vi "createTable sortie ROI.vi"() -> ()   [LabVIEW 2019]
panel:
  out "R7 chiffre":string
  out "R1 chiffre":string
  out "R4 chiffre":string
  out "Y3 chiffre":string
  out "Y1 chiffre":string
  out "Y2 chiffre":string
  out "G6 chiffre":string
  out "G9 chiffre":string
  out "Y7 chiffre":string
  out "R2 chiffre":string
  out "Y4 chiffre":string
  out "G3 chiffre":string
  out "G7 chiffre":string
  out "O3 chiffre":string
  out "G2 chiffre":string
  out "O9 chiffre":string
  out "W7 chiffre":string
  out "W8 chiffre":string
  out "W9 chiffre":string
  out "G8 chiffre":string
  out "G4 chiffre":string
  out "O6 chiffre":string
  out "G1 chiffre":string
  out "W6 chiffre":string
  out "O2 chiffre":string
  out "O1 chiffre":string
  out "O8 chiffre":string
  out "O7 chiffre":string
  out "O4 chiffre":string
  out "Y6 chiffre":string
  out "Y8 chiffre":string
  out "Y9 chiffre":string
  out "B7 chiffre":string
  out "B4 chiffre":string
  out "R8 chiffre":string
  out "B2 chiffre":string
  out "W4 chiffre":string
  out "R9 chiffre":string
  out "B8 chiffre":string
  out "B9 chiffre":string
  out "B6 chiffre":string
  out "R3 chiffre":string
  out "B3 chiffre":string
  out "B1 chiffre":string
  out "W3 chiffre":string
  out "R6 chiffre":string
  out "W2 chiffre":string
  out "W1 chiffre":string
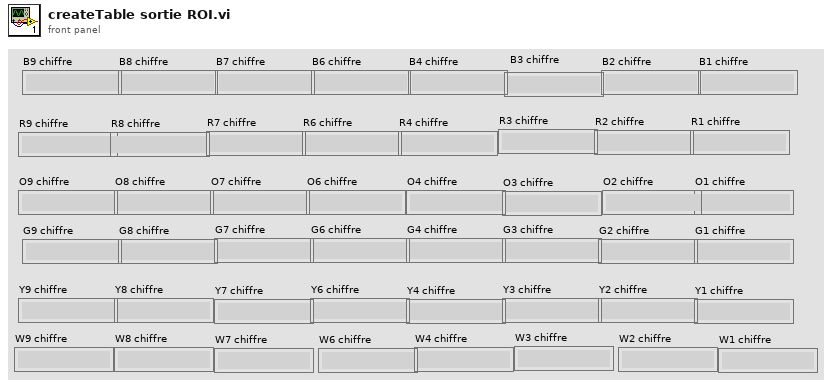
[diagram p1: front panel]
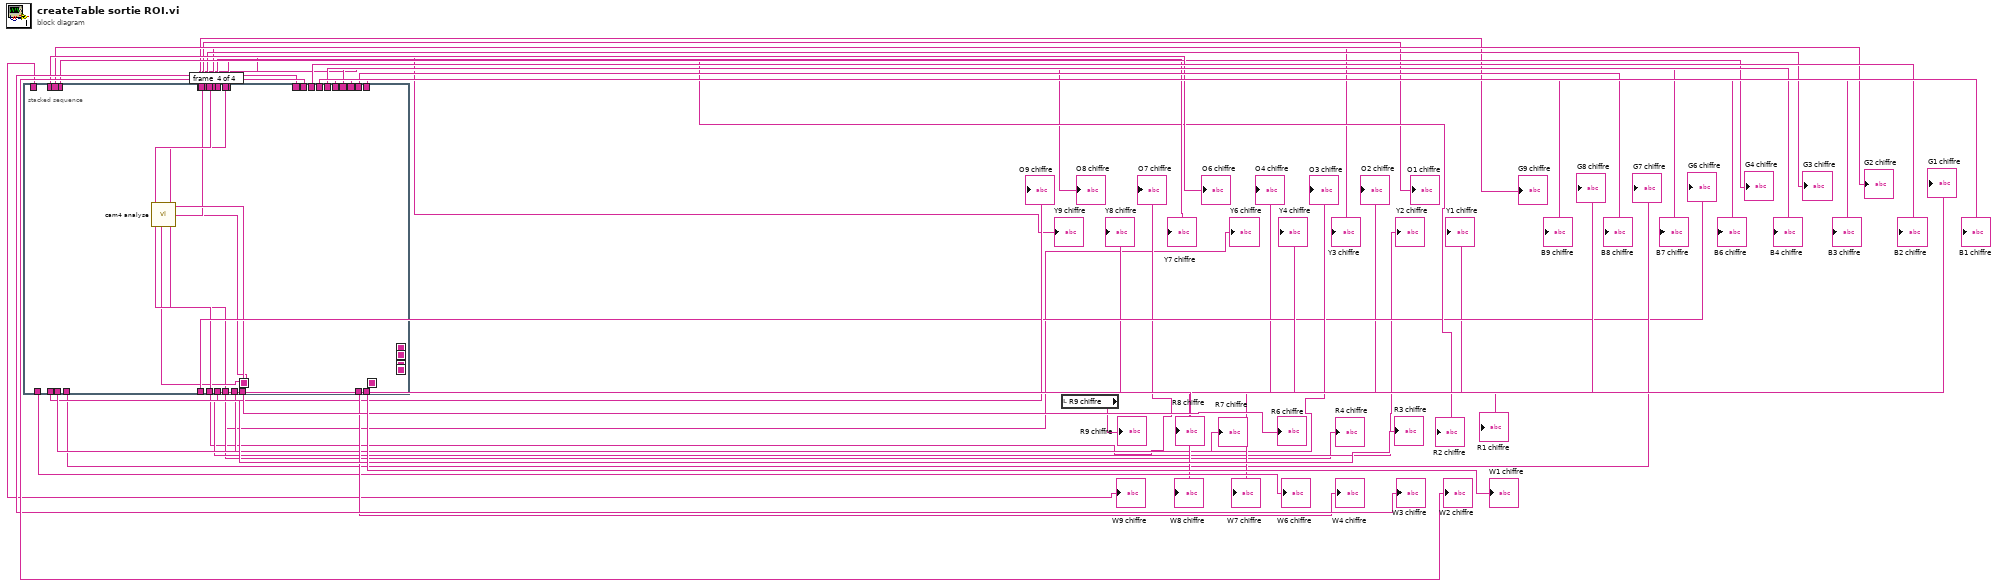
[diagram p0: block diagram]
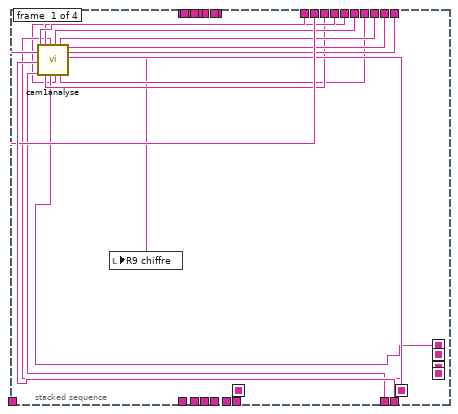
[diagram p2: hidden frame]
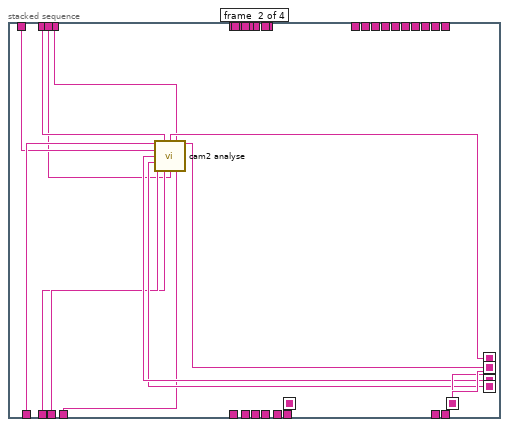
[diagram p3: hidden frame]
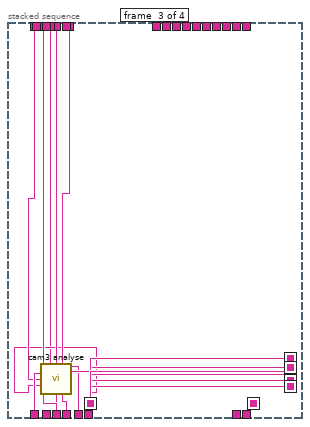
[diagram p4: hidden frame]
diagram:
  n1 = stacked-sequence {
    seq-local: [w62 _ _ _] -> [_ w79 _ _]
    seq-local: [w58 _ _ _] -> [_ w78 _ _]
    seq-local: [w52 _ _ _] -> [_ w77 _ _]
    seq-local: [_ w79 _ _] -> [_ _ w98 _]
    seq-local: [_ w78 _ _] -> [_ _ w97 _]
    seq-local: [_ w77 _ _] -> [_ _ w96 _]
    seq-local: [_ w74 _ _] -> [_ _ w95 _]
    seq-local: [_ w72 _ _] -> [_ _ w94 _]
    seq-local: [_ w70 _ _] -> [_ _ w93 _]
    seq-local: [_ w69 _ _] -> [_ _ w92 _]
    seq-local: [_ _ w98 _] -> [_ _ _ w115]
    seq-local: [_ _ w97 _] -> [_ _ _ w114]
    seq-local: [_ _ w96 _] -> [_ _ _ w113]
    seq-local: [_ _ w95 _] -> [_ _ _ w112]
    seq-local: [_ _ w94 _] -> [_ _ _ w111]
    seq-local: [_ _ w93 _] -> [_ _ _ w110]
    seq-local: [_ _ w92 _] -> [_ _ _ w109]
    seq-local: [_ _ w90 _] -> [_ _ _ w108]
    seq-local: [_ _ w84 _] -> [_ _ _ w107]
    tunnel: [w64 _ _ _] -> w48
    tunnel: [w63 _ _ _] -> w47
    tunnel: [w61 _ _ _] -> w45
    tunnel: [w60 _ _ _] -> w44
    tunnel: [w59 _ _ _] -> w43
    tunnel: [w57 _ _ _] -> w41
    tunnel: [w56 _ _ _] -> w40
    tunnel: [w55 _ _ _] -> w39
    tunnel: [w54 _ _ _] -> w38
    tunnel: [w53 _ _ _] -> w37
    tunnel: [w51 _ _ _] -> w35
    tunnel: [w50 _ _ _] -> w34
    tunnel: [_ w76 _ _] -> w33
    tunnel: [_ w75 _ _] -> w32
    tunnel: [_ w73 _ _] -> w30
    tunnel: [_ w71 _ _] -> w28
    tunnel: [_ w68 _ _] -> w25
    tunnel: [_ w67 _ _] -> w24
    tunnel: [_ w66 _ _] -> w23
    tunnel: [_ w65 _ _] -> w22
    tunnel: [_ _ w91 _] -> w21
    tunnel: [_ _ w89 _] -> w19
    tunnel: [_ _ w88 _] -> w18
    tunnel: [_ _ w87 _] -> w17
    tunnel: [_ _ w86 _] -> w16
    tunnel: [_ _ w85 _] -> w15
    tunnel: [_ _ w83 _] -> w13
    tunnel: [_ _ w82 _] -> w12
    tunnel: [_ _ w81 _] -> w11
    tunnel: [_ _ w80 _] -> w10
    tunnel: [_ _ _ w115] -> w46
    tunnel: [_ _ _ w114] -> w42
    tunnel: [_ _ _ w113] -> w36
    tunnel: [_ _ _ w112] -> w31
    tunnel: [_ _ _ w111] -> w29
    tunnel: [_ _ _ w110] -> w27
    tunnel: [_ _ _ w109] -> w26
    tunnel: [_ _ _ w108] -> w20
    tunnel: [_ _ _ w107] -> w14
    tunnel: [_ _ _ w106] -> w9
    tunnel: [_ _ _ w105] -> w8
    tunnel: [_ _ _ w104] -> w7
    tunnel: [_ _ _ w103] -> w6
    tunnel: [_ _ _ w102] -> w5
    tunnel: [_ _ _ w101] -> w4
    tunnel: [_ _ _ w100] -> w3
    tunnel: [_ _ _ w99] -> w2
    frame #0 {
      n2 = call "cam1analyse.vi"() -> ("W3 chiffre"=w61:string, "W2 chiffre"=w63:string, "R6 chiffre"=w62:string, "W1 chiffre"=w64:string, "W4 chiffre"=w54:string, "B1 chiffre"=w60:string, "B2 chiffre"=w53:string, "R3 chiffre"=w58:string, "R8 chiffre"=w52:string, "B3 chiffre"=w59:string, "B4 chiffre"=w51:string, "B6 chiffre"=w57:string, "B7 chiffre"=w50:string, "B8 chiffre"=w55:string, "B9 chiffre"=w56:string, "R9 chiffre"=w49:string)  [unwired: 4 in]
      n3 = local write "R9 chiffre"(w49) -> ()
    }
    frame #1 {
      n4 = call "cam2 analyse.vi"() -> ("W6 chiffre"=w76:string, "O6 chiffre"=w75:string, "G1 chiffre"=w74:string, "G4 chiffre"=w73:string, "G8 chiffre"=w72:string, "W9 chiffre"=w71:string, "W8 chiffre"=w70:string, "W7 chiffre"=w69:string, "O3 chiffre"=w68:string, "O9 chiffre"=w67:string, "G2 chiffre"=w66:string, "G7 chiffre"=w65:string)  [unwired: 4 in]
    }
    frame #2 {
      n5 = call "cam3 analyse.vi"() -> ("G3 chiffre"=w91:string, "Y4 chiffre"=w90:string, "Y7 chiffre"=w89:string, "R2 chiffre"=w88:string, "R7 chiffre"=w87:string, "G6 chiffre"=w86:string, "G9 chiffre"=w85:string, "Y1 chiffre"=w84:string, "Y2 chiffre"=w83:string, "Y3 chiffre"=w82:string, "R1 chiffre"=w81:string, "R4 chiffre"=w80:string)  [unwired: 4 in]
    }
    frame #3 {
      n6 = call "cam4 analyse.vi"() -> ("O1 chiffre"=w106:string, "O2 chiffre"=w105:string, "O8 chiffre"=w104:string, "O7 chiffre"=w103:string, "O4 chiffre"=w102:string, "Y9 chiffre"=w101:string, "Y8 chiffre"=w100:string, "Y6 chiffre"=w99:string)
    }
  }
  "W1 chiffre" <- w48
  "W2 chiffre" <- w47
  "R6 chiffre" <- w46
  "W3 chiffre" <- w45
  "B1 chiffre" <- w44
  "B3 chiffre" <- w43
  "R3 chiffre" <- w42
  "B6 chiffre" <- w41
  "B9 chiffre" <- w40
  "B8 chiffre" <- w39
  "W4 chiffre" <- w38
  "B2 chiffre" <- w37
  "R8 chiffre" <- w36
  "B4 chiffre" <- w35
  "B7 chiffre" <- w34
  "Y9 chiffre" <- w4
  "Y8 chiffre" <- w3
  "Y6 chiffre" <- w2
  "O4 chiffre" <- w5
  "O7 chiffre" <- w6
  "O8 chiffre" <- w7
  "O1 chiffre" <- w9
  "O2 chiffre" <- w8
  "W6 chiffre" <- w33
  "G1 chiffre" <- w31
  "O6 chiffre" <- w32
  "G4 chiffre" <- w30
  "G8 chiffre" <- w29
  "W9 chiffre" <- w28
  "W8 chiffre" <- w27
  "W7 chiffre" <- w26
  "O9 chiffre" <- w24
  "G2 chiffre" <- w23
  "O3 chiffre" <- w25
  "G7 chiffre" <- w22
  "G3 chiffre" <- w21
  "Y4 chiffre" <- w20
  "R2 chiffre" <- w18
  "Y7 chiffre" <- w19
  "G9 chiffre" <- w15
  "G6 chiffre" <- w16
  "Y2 chiffre" <- w13
  "Y1 chiffre" <- w14
  "Y3 chiffre" <- w12
  "R4 chiffre" <- w10
  "R1 chiffre" <- w11
  "R7 chiffre" <- w17
  n7 = local read "R9 chiffre"() -> (→"R9 chiffre":string)
